vi "Dictionary Get Data__ogtk.vi"(8 "error in (no error)":errorcluster, 11 "Object RefNum":T1) -> (0 "error out":errorcluster, 2 "Data out":T2, 3 "Dup Object RefNum":T1)   [LabVIEW 2012]
doc: "Gets the GOOP data structure without mutex"
uses:
  <userlib>/_OpenG.lib/dictionary/dictionary.llb/Dictionary Data__ogtk.ctl
  <userlib>/_OpenG.lib/dictionary/dictionary.llb/Dictionary Object RefNum__ogtk.ctl
  <userlib>/_OpenG.lib/dictionary/dictionary.llb/Dictionary Object RefNum - Enum__ogtk.ctl
  <userlib>/_OpenG.lib/dictionary/dictionary.llb/Dictionary Object Data Core Task Enum__ogtk.ctl
panel:
  # "OpenGOOP Get Data.vi\n\nGets the GOOP data structure without mutex\n\nPlease visit http://www.OpenG.org to learn about the\nOpen Source LabVIEW software movement.\n\nNOTICE -- YOU MUST LEAVE THIS NOTICE IN PLACE.  PER THE TERMS OF THE LICENSE BELOW, YOU MAY SUBLICENSE THIS SOFTWARE \nIN ANY WAY THAT DOES NOT CONFLICT WITH THIS LICENSE.\n\n### BSD License (http://www.opensource.org/licenses/bsd-license.php) Begin ###\n \nCopyright (c) 2002, Jim Kring <jim@jimkring.com>\n\nAll rights reserved.\n\nRedistribution and use in source and binary forms, with or without modification, are permitted provided that the following conditions are met:\n\n    * Redistributions of source code must retain the above copyright notice, this list of conditions and the following disclaimer.\n    * Redistributions in binary form must reproduce the above copyright notice, this list of conditions and the following disclaimer in the \n       documentation and/or other materials provided with the distribution.\n    * Neither the name of SciWare, James Kring, Inc., nor the names of its contributors may be used to endorse or promote products derived \n       from this software without specific prior written permission.\n\nTHIS SOFTWARE IS PROVIDED BY THE COPYRIGHT HOLDERS AND CONTRIBUTORS \"AS IS\" AND ANY EXPRESS OR IMPLIED WARRANTIES, \nINCLUDING, BUT NOT LIMITED TO, THE IMPLIED WARRANTIES OF MERCHANTABILITY AND FITNESS FOR A PARTICULAR PURPOSE ARE \nDISCLAIMED. IN NO EVENT SHALL THE COPYRIGHT OWNER OR CONTRIBUTORS BE LIABLE FOR ANY DIRECT, INDIRECT, INCIDENTAL,\n SPECIAL, EXEMPLARY, OR CONSEQUENTIAL DAMAGES (INCLUDING, BUT NOT LIMITED TO, PROCUREMENT OF SUBSTITUTE GOODS OR \nSERVICES; LOSS OF USE, DATA, OR PROFITS; OR BUSINESS INTERRUPTION) HOWEVER CAUSED AND ON ANY THEORY OF LIABILITY, \nWHETHER IN CONTRACT, STRICT LIABILITY, OR TORT (INCLUDING NEGLIGENCE OR OTHERWISE) ARISING IN ANY WAY OUT OF THE USE \nOF THIS SOFTWARE, EVEN IF ADVISED OF THE POSSIBILITY OF SUCH DAMAGE.\n\n### BSD License End ###"
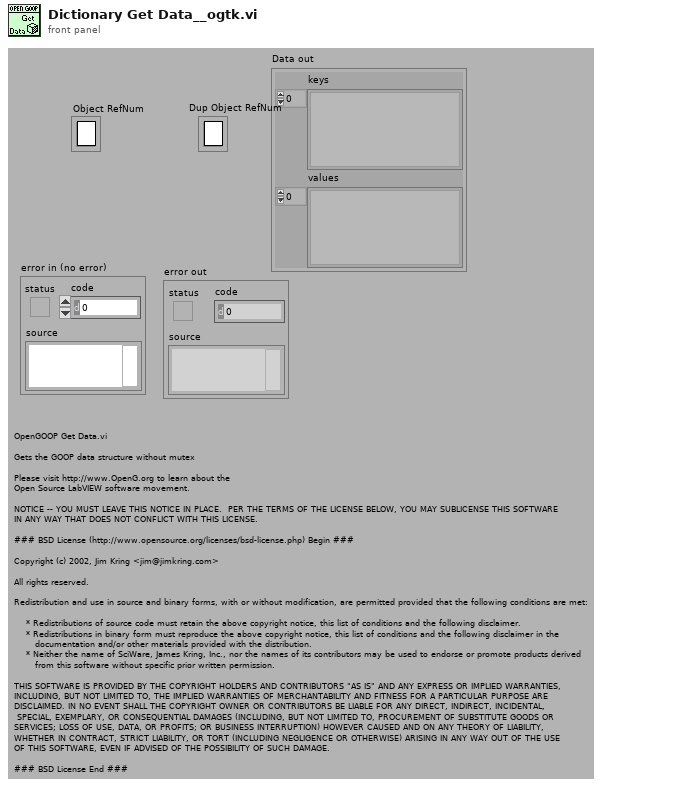
[diagram p1: front panel]
types:
  T1 = typedef "Dictionary Object RefNum__ogtk.ctl" = refnum<k1>
  T2 = typedef "Dictionary Data__ogtk.ctl" = cluster{"keys":variant[], "values":variant[]}
  T3 = typedef "Dictionary Object Data Core Task Enum__ogtk.ctl" = enum16{"read", "write", "init"}
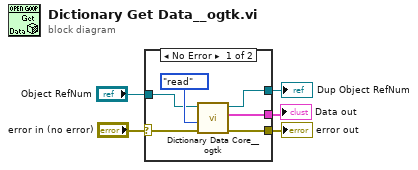
[diagram p0: block diagram]
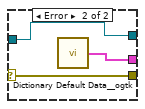
[diagram p2: hidden frame]
diagram:
  n1 = case shown="No Error" "error in (no error)" {
    selector: "error in (no error)" -> [w10 w14]
    tunnel: [w11 w14] -> w5
    tunnel: [w8 w13] -> w3
    tunnel: [w7 w12] -> w2
    tunnel: "Object RefNum" -> [w6 w12]
    frame No Error {
      n2 = call <userlib>:"Dictionary Data Core__ogtk.vi"("error in (no error)"=w10, "task (read)"=Dictionary_Object_Data_Core_Task_Enum__ogtk."read", "Object RefNum"=w6) -> ("error out"=w11:errorcluster, "Data out"=w8:T2, "dup Object RefNum"=w7:T1)  [unwired: 6 in]
    }
    frame Error {
      n3 = call <userlib>:"Dictionary Default Data__ogtk.vi"() -> ("Data out"=w13:T2)
    }
  }
  "error out" <- w5
  "Data out" <- w3
  "Dup Object RefNum" <- w2
